vi "UnitToValue.vi"(10 "unit":string, 11 "value in":dbl) -> (3 "value out":dbl)   [LabVIEW 2018, in "Library-DataConvert.lvlib"]
uses:
  Library-DataConvert.lvlib
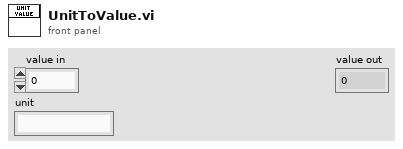
[diagram p1: front panel]
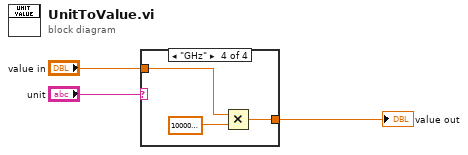
[diagram p0: block diagram]
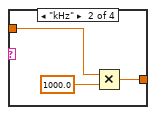
[diagram p3: hidden frame]
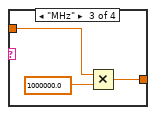
[diagram p4: hidden frame]
diagram:
  n1 = case shown="\"GHz\"" "unit" {
    tunnel: [w4 w6 w9 w12] -> w1
    tunnel: "value in" -> [w4 w5 w8 w11]
    frame Default {
    }
    frame "kHz" {
      n2 = Multiply(x=w5, y=1000.0) -> (x*y=w6:dbl)
    }
    frame "MHz" {
      n3 = Multiply(x=w8, y=1000000.0) -> (x*y=w9:dbl)
    }
    frame "GHz" {
      n4 = Multiply(x=w11, y=1000000000.0) -> (x*y=w12:dbl)
    }
  }
  "value out" <- w1
